vi "JKISM++ Get New State Notifier Event.vi"(8 "Error in":errorcluster caption="Error in (no error)", 11 "Name(\"\" to use uuid) in":string) -> (0 "Error out":errorcluster, 3 "New State Notifier Event":refnum<user-event>)   [LabVIEW 2014, in "JKI State Machine++.lvlib"]
doc: "<b>Inputs:</b>\n - <b>Name(\"\" to use uuid) in</b>: JKISM module name\n - <b>Error in</b>: Error cluster\n\n<b>Outputs:</b>\n - <b>New State Notifier Event</b>: User event to break JKISM module from waiting in event structure when message is received.\n - <b>Error out</b>: Error cluster"
uses:
  JKI State Machine++.lvlib
  _Support/JKISMQ/_JKISMQFGVOPER.ctl
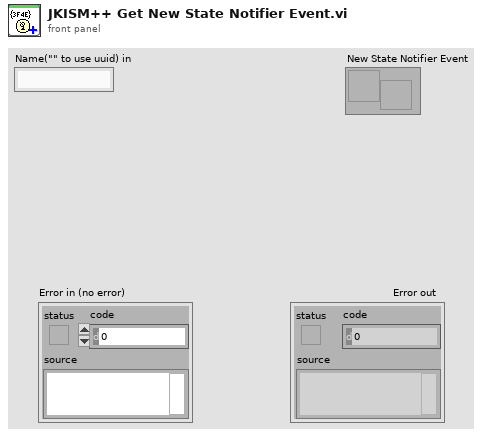
[diagram p1: front panel]
types:
  T1 = typedef "JKI State Machine++.lvlib/_JKISMQFGVOPER.ctl" = enum16{"Get By Name", "List", "Check If Name Exists", "Release", "Module Status"}
  T2 = typedef "JKI State Machine++.lvlib/_JKISMQ.ctl" = cluster{"Module Name":string, "Queue":refnum<queue>, "Locked Status":refnum<data-value>, "Mode":T3, "User Event":refnum<user-event>, "Queue Count":i32}
  T3 = typedef "JKI State Machine++.lvlib/_JKISM_MODE.ctl" = enum16{"Stand Alone", "JKISM", "Action Worker"}
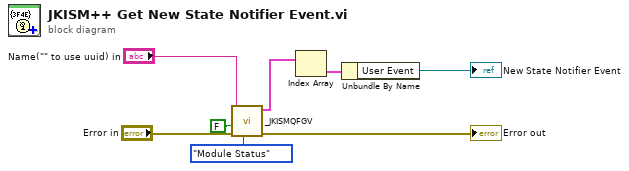
[diagram p0: block diagram]
diagram:
  n1 = call "_JKISMQFGV.vi"("Operation"=_JKISMQFGVOPER."Module Status", "Error in"="Error in", "create if not found? (T)"=FALSE, "Name(\"\" to use uuid) in"="Name(\"\" to use uuid) in") -> ("Error out"=→"Error out":errorcluster, "Array"=w3:T2[])  [unwired: 4 in, 2 out]
  n2 = Index Array(array=w3) -> (element=w2:T2)  [unwired: 1 in]
  n3 = Unbundle By Name(w2) -> ("User Event"=→"New State Notifier Event":refnum<user-event>)
